vi "Close Module.vi"(8 "error in (no error)":errorcluster, 9 "Wait for stop?":bool, 11 "Module Admin in":refnum<class "Delacor_lib_QMH_Cloneable Module Admin.lvclass">) -> (0 "error out":errorcluster, 1 "External Launch":bool, 3 "Module Admin out":refnum<class "Delacor_lib_QMH_Cloneable Module Admin.lvclass">)   [LabVIEW 2015, in "ISA010_module.lvlib"]
doc: "Destroy the Broadcast Events and Request Events (if this was the first instance). Reset flags stored in Module Admin class.\n_____\nBased on Delacor QMH Project Template 3.1.0.34."
uses:
  ISA010_module.lvlib
  <vilib>/Delacor/Delacor QMH/Libraries/Cloneable Module Admin_class/Delacor_lib_QMH_Cloneable Module Admin.lvclass
  <vilib>/Delacor/Delacor QMH/Libraries/Cloneable Module Admin_class/Delacor_lib_QMH_Cloneable Module Admin.lvclass/Delacor_lib_QMH_Cloneable Module Admin.ctl
  <vilib>/Delacor/Delacor QMH/Libraries/Module Admin_class/Delacor_lib_QMH_Module Admin.lvclass/Delacor_lib_QMH_Module Admin.ctl
  <vilib>/Delacor/Delacor QMH/Libraries/Cloneable Module Admin_class/Delacor_lib_QMH_Get First.vi
  <vilib>/Delacor/Delacor QMH/Libraries/Cloneable Module Admin_class/Delacor_lib_QMH_Get Module ID.vi
  <vilib>/Delacor/Delacor QMH/Libraries/Module Admin_class/Delacor_lib_QMH_Get External Launch.vi
  Clone Registration/Clone Registration.lvlib
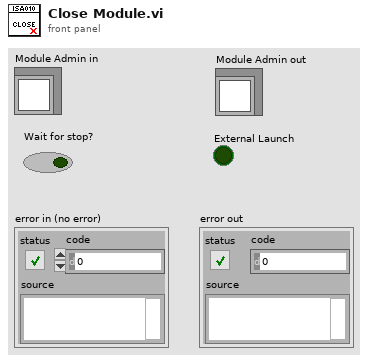
[diagram p1: front panel]
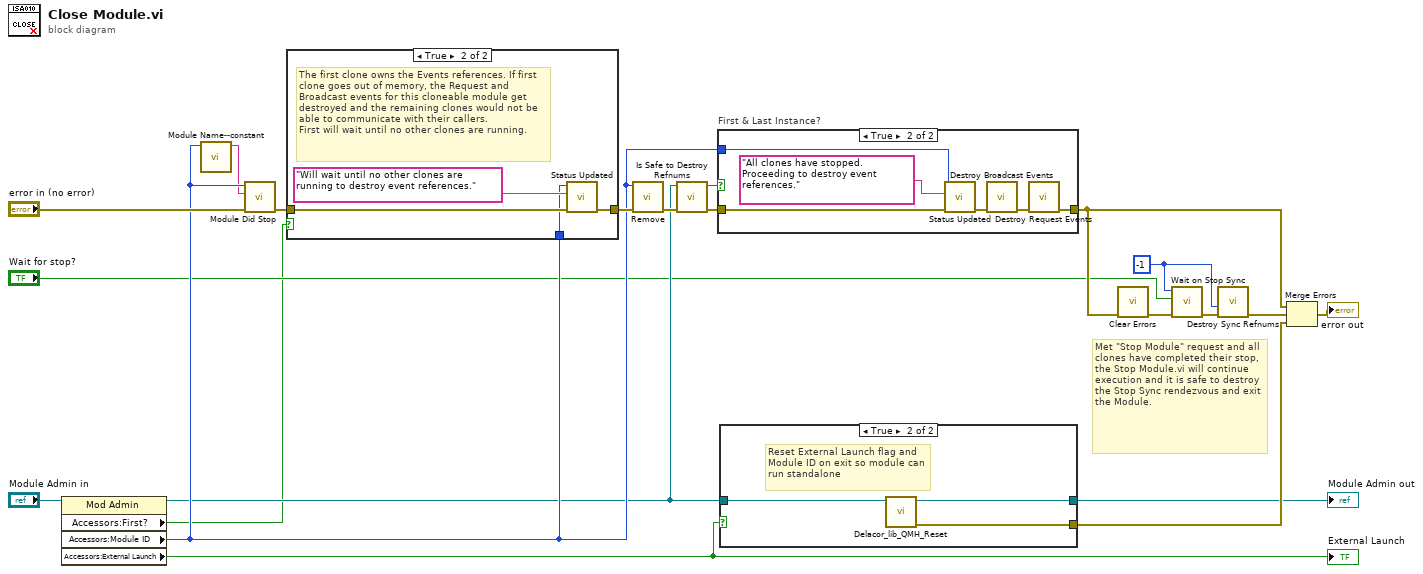
[diagram p0: block diagram]
diagram:
  w6 = -1 ("Module ID")
  # "Met \"Stop Module\" request and all clones have completed their stop, the Stop Module.vi will continue execution and it is safe to destroy the Stop Sync rendezvous and exit the Module."
  n1 = property class="Mod Admin"(reference="Module Admin in") -> (reference out=w15:refnum<class "Delacor_lib_QMH_Cloneable Module Admin.lvclass">, "Accessors:First?"=w3:bool, "Accessors:Module ID"=w19:i32, "Accessors:External Launch"=w2:bool)  [unwired: 1 in, 1 out]
  "External Launch" <- w2
  n2 = call "Module Name--constant.vi"("Module ID"=w19) -> ("Module Name"=w1:string)  [unwired: 10 in]
  n3 = call "Module Did Stop.vi"("error in (no error)"="error in (no error)", "Origin"=w1, "Module ID"=w19) -> ("error out"=w10:errorcluster)  [unwired: 8 in]
  n4 = case shown="True" w3 {
    tunnel: w10 -> [w22 w26]
    tunnel: w19 -> [_ w24]
    tunnel: [w22 w23] -> w21
    frame False {
    }
    frame True {
      # "The first clone owns the Events references. If first clone goes out of memory, the Request and Broadcast events for this cloneable module get destroyed and the remaining clones would not be able to communicate with their callers.\nFirst will wait until no other clones are running."
      n5 = call "Status Updated.vi"("error in (no error)"=w26, "Status"="Will wait until no other clones are running to destroy event references." ("format string"), "Module ID"=w24) -> ("error out"=w23:errorcluster)  [unwired: 8 in]
    }
  }
  n6 = call "Remove.vi"("error in (no error)"=w21, "Module ID"=w19) -> ("error out"=w16:errorcluster)  [unwired: 8 in, 1 out]
  n7 = call "Is Safe to Destroy Refnums.vi"("error in (no error)"=w16, "Module Admin"=w15) -> ("error out"=w12:errorcluster, "Destroy Broadcast & Request Event Refs?"=w13:bool)  [unwired: 8 in]
  n8 = case "First & Last Instance?" shown="True" w13 {
    tunnel: w12 -> [w27 w31]
    tunnel: [w27 w33] -> w18
    tunnel: w19 -> [_ w29]
    frame False {
    }
    frame True {
      n9 = call "Status Updated.vi"("error in (no error)"=w31, "Status"="All clones have stopped. Proceeding to destroy event references.", "Module ID"=w29) -> ("error out"=w30:errorcluster)  [unwired: 8 in]
      n10 = call "Destroy Broadcast Events.vi"("error in (no error)"=w30) -> ("error out"=w32:errorcluster)  [unwired: 10 in]
      n11 = call "Destroy Request Events.vi"("error in (no error)"=w32) -> ("error out"=w33:errorcluster)  [unwired: 10 in]
    }
  }
  n12 = case shown="True" w2 {
    tunnel: w15 -> [w34 w37]
    tunnel: [w34 w36] -> w11
    tunnel: [_ w35] -> w17
    frame False {
    }
    frame True {
      # "Reset External Launch flag and Module ID on exit so module can run standalone"
      n13 = call-dynamic "Delacor_lib_QMH_Reset.vi"("Mod Admin in"=w37) -> ("error out"=w35:errorcluster, "Mod Admin out"=w36:refnum<class "Delacor_lib_QMH_Cloneable Module Admin.lvclass">)  [unwired: 9 in]
    }
  }
  "Module Admin out" <- w11
  n14 = call <vilib>:"Clear Errors.vi"("error in (no error)"=w18) -> ("error out"=w5:errorcluster)  [unwired: 5 in, 1 out]
  n15 = call "Wait on Stop Sync.vi"("error in (no error)"=w5, "Wait for Module to stop?"="Wait for stop?", "Module ID"=w6) -> ("error out"=w9:errorcluster)  [unwired: 8 in]
  n16 = call "Destroy Sync Refnums.vi"("error in (no error)"=w9, "Module ID"=w6) -> ("error out"=w7:errorcluster)  [unwired: 9 in]
  n17 = Merge Errors(w18, w7, w17) -> (→"error out":errorcluster)
